vi "Get U64 Package Attribute Value.vi"(8 "error in (no error)":errorcluster, 10 "package attribute name":string, 11 "package attributes CLI string":string) -> (0 "error out":errorcluster, 3 "package attribute value":u64)   [LabVIEW 2014, in "NIPM_API.lvlib"]
uses:
  NIPM_API.lvlib
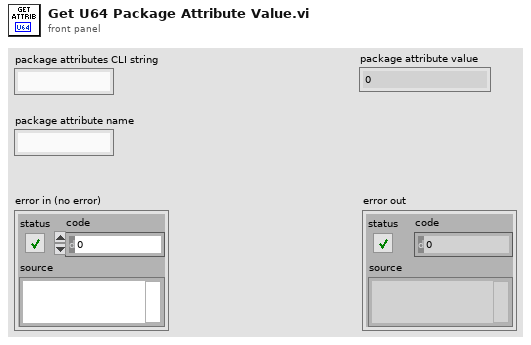
[diagram p1: front panel]
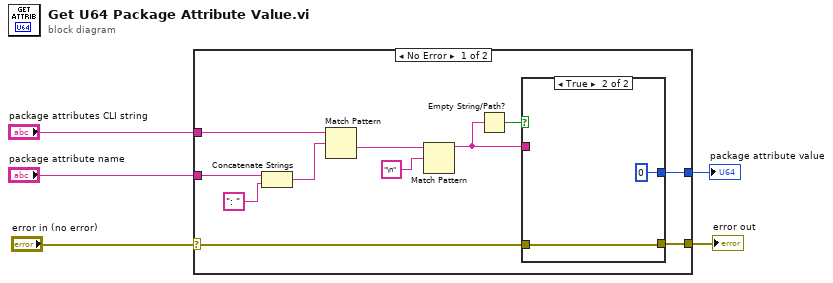
[diagram p0: block diagram]
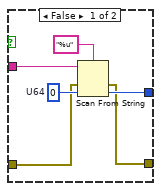
[diagram p2: hidden frame]
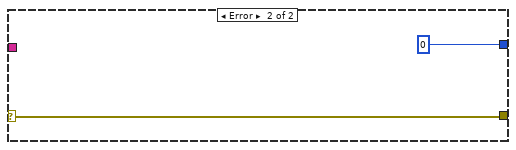
[diagram p3: hidden frame]
diagram:
  n1 = case shown="No Error" "error in (no error)" {
    selector: "error in (no error)" -> [w8 w25]
    tunnel: "package attribute name" -> [w14 _]
    tunnel: "package attributes CLI string" -> [w13 _]
    tunnel: [w10 u64 0 ("U64")] -> w3
    tunnel: [w7 w25] -> w1
    frame No Error {
      n2 = Concatenate Strings(w14, ": " ("string")) -> (w12:string)
      n3 = Match Pattern(string=w13, regular expression=w12) -> (after substring=w15:string)  [unwired: 1 in, 3 out]
      n4 = Match Pattern(string=w15, regular expression="\n") -> (before substring=w9:string)  [unwired: 1 in, 3 out]
      n5 = Empty String/Path?(string/path=w9) -> (empty?=w6:bool)
      n6 = case shown="True" w6 {
        tunnel: [w20 u64 0 ("U64")] -> w10
        tunnel: w9 -> [w19 _]
        tunnel: w8 -> [w18 w23]
        tunnel: [w17 w23] -> w7
        frame False {
          w21 = u64 0  # U64
          n7 = Scan From String(format string="%u", input string=w19, error in=w18, default 1=w21) -> (error out=w17:errorcluster, output 1=w20:u64)  [unwired: 1 in, 2 out]
        }
        frame True {
        }
      }
    }
    frame Error {
    }
  }
  "package attribute value" <- w3
  "error out" <- w1
